vi "DAQmxTerminalTest.vi"() -> ()   [LabVIEW 2014, in "FGenModule.lvlib"]
uses:
  FGenModule/FGenModule.lvlib
  <resource>/objmgr/daqmx.rc
  <vilib>/Instr/_visa.llb/VISA Find Search Mode.ctl
  <instrlib>/niSync/niSync.llb/niSync Initialize (IVI).vi
panel:
  out "String 2":string
  out "Array 2":string[](array[string])
  out "String":string
  out "Array":string[][](array[string])
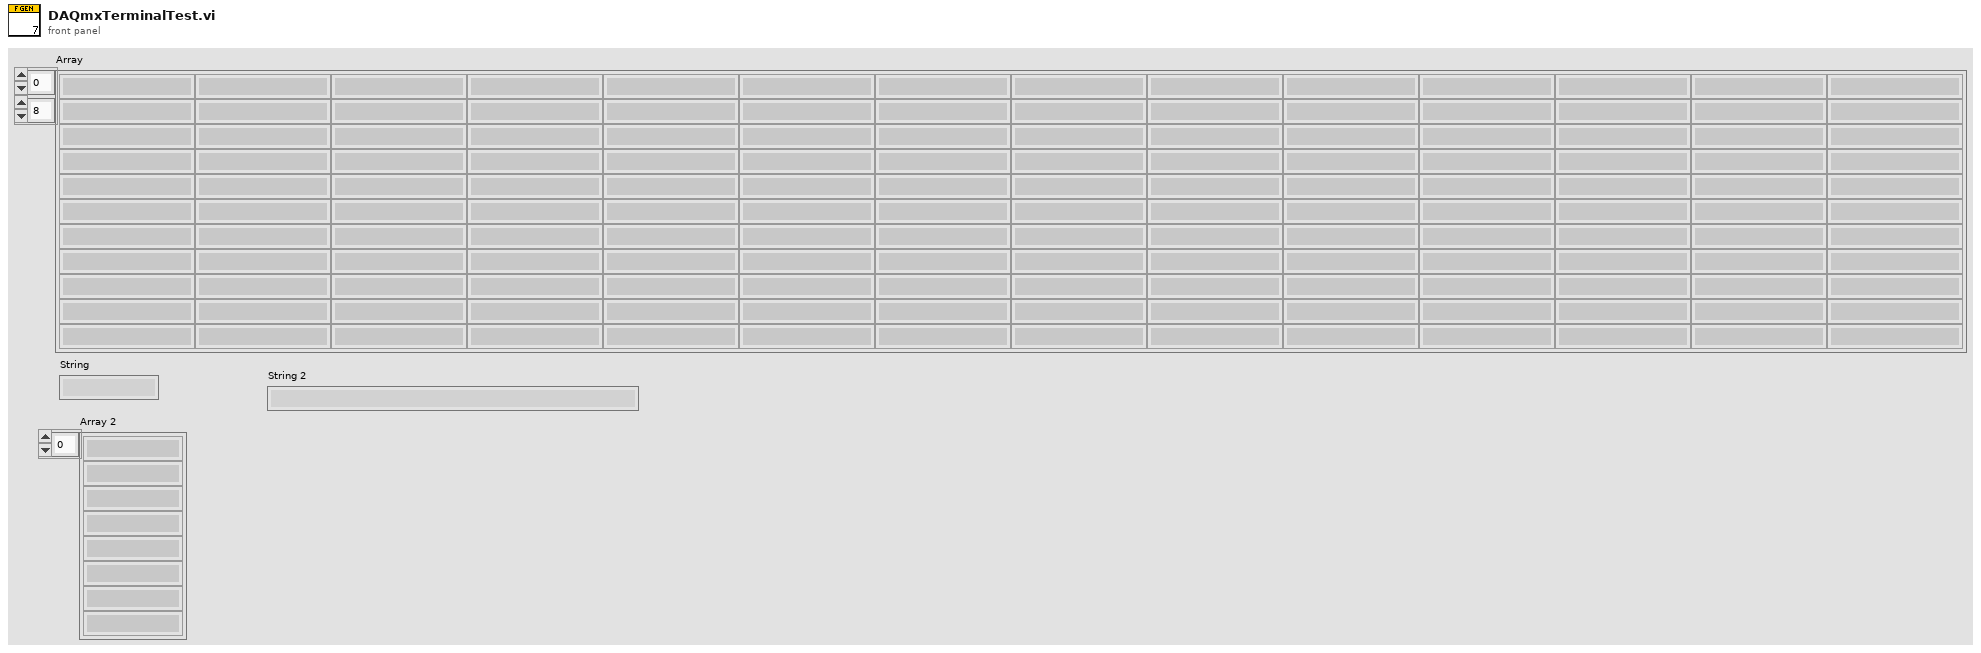
[diagram p1: front panel]
types:
  T1 = typedef "VISA Find Search Mode.ctl" = u32
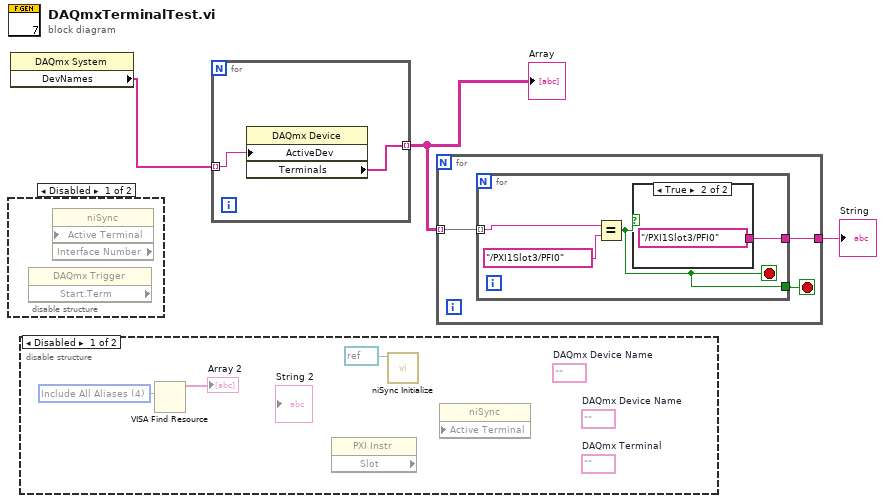
[diagram p0: block diagram]
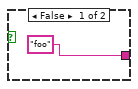
[diagram p4: hidden frame]
diagram:
  n1 = disable-structure shown="Disabled" {
    frame Disabled {
      n2 = property class="DAQmx Trigger" props=["Start.Term"]() -> ()  [unwired: 2 in, 3 out]
      n3 = property class="niSync" props=["Active Terminal", "Interface Number"]() -> ()  [unwired: 3 in, 3 out]
    }
    frame Enabled {
    }
  }
  n4 = property on="Property Node" class="DAQmx System"() -> ("DevNames"=w3:tag[])  [unwired: 2 in, 2 out]
  n5 = disable-structure shown="Disabled" {
    frame Disabled {
      (unwired) tag ""  # DAQmx Device Name
      (unwired) tag ""  # DAQmx Terminal
      w5 = T1 4 items=["Canonical Names Only"=0, "Aliases Only"=2, "Include Matching Aliases"=3, "Include All Aliases"=4] ("Search Mode")
      (unwired) tag ""  # DAQmx Device Name
      n6 = VISA Find Resource(10:w5) -> (3:→"Array 2":string[])  [unwired: 2 in, 2 out]
      n7 = property class="PXI Instr" props=["Slot"]() -> ()  [unwired: 2 in, 3 out]
      n8 = call-poly <instrlib>:"niSync Initialize.vi"("resource name"=refnum<k15> refnum) -> ()  [unwired: 9 in, 2 out]
      n9 = property class="niSync" props=["Active Terminal"]() -> ()  [unwired: 3 in, 2 out]
    }
    frame Enabled {
    }
  }
  n10 = for {
    tunnel: w3 -> [w7] mode=indexing
    tunnel: [w8] -> w2 mode=indexing
    n11 = property class="DAQmx Device"("ActiveDev"=w7) -> ("Terminals"=w8:tag[])  [unwired: 2 in, 2 out]
  }
  "Array" <- w2
  n12 = for {
    tunnel: w2 -> [w11] mode=indexing
    tunnel: [w9] -> w1
    stop <- w10 stop-if-true
    n13 = for {
      tunnel: w11 -> [w15] mode=indexing
      tunnel: [w13] -> w10
      tunnel: [w12] -> w9
      stop <- w13 stop-if-true
      n14 = Equal?(x=w15, y=tag "/PXI1Slot3/PFI0" ("source")) -> (x = y?=w13:bool)
      n15 = case shown="True" w13 {
        tunnel: ["foo" tag "/PXI1Slot3/PFI0" ("source")] -> w12
        frame False {
        }
        frame True {
        }
      }
    }
  }
  "String" <- w1
